vi "testCreateQueues.vi"(8 "error in (no error)":errorcluster) -> (0 "error out":errorcluster)   [LabVIEW 2018]
doc: "Test the createQueues.vi."
uses:
  src/TcpServerBase/TcpServerBase.lvclass
  src/TcpServerBase/TcpServerBase.lvclass/TcpServerBase.ctl
  <vilib>/addons/_JKI Toolkits/Caraya/classes/Assert/Assert Equal Type_Variant.vi
  <vilib>/addons/_JKI Toolkits/Caraya/classes/Test/Test.lvclass
  <vilib>/addons/_JKI Toolkits/Caraya/classes/Assert/Assert.lvclass
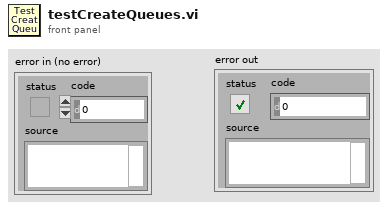
[diagram p1: front panel]
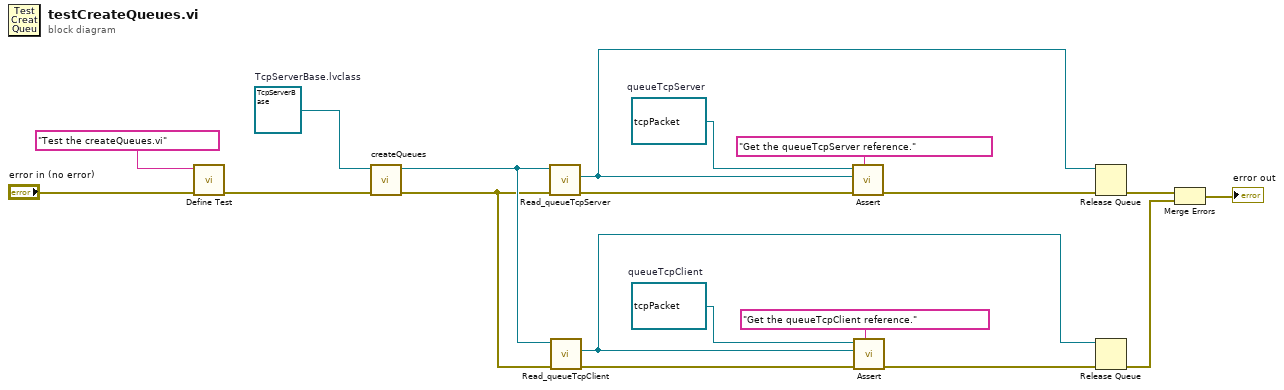
[diagram p0: block diagram]
diagram:
  w1 = refnum<queue> refnum  # queueTcpClient
  w2 = refnum<queue> refnum  # queueTcpServer
  w12 = refnum<class "TcpServerBase.lvclass"> refnum  # TcpServerBase.lvclass
  n1 = call <vilib>:"Define Test.vi"("error in (no error)"="error in (no error)", "Label (VI Title)"="Test the createQueues.vi") -> ("error out"=w11:errorcluster)  [unwired: 9 in]
  n2 = call "createQueues.vi"("error in (no error)"=w11, "tcpServerBase in"=w12) -> ("error out"=w9:errorcluster, "tcpServerBase out"=w10:refnum<class "TcpServerBase.lvclass">)  [unwired: 8 in]
  n3 = call "Read_queueTcpServer.vi"("error in (no error)"=w9, "TcpServerBase in"=w10) -> ("error out"=w8:errorcluster, "queueTcpServer"=w4:refnum<queue>)  [unwired: 7 in, 1 out]
  n4 = call "Read_queueTcpClient.vi"("error in (no error)"=w9, "TcpServerBase in"=w10) -> ("error out"=w7:errorcluster, "queueTcpClient"=w3:refnum<queue>)  [unwired: 7 in, 1 out]
  n5 = call-poly <vilib>:"Assert.vi"("Label"="Get the queueTcpServer reference.", "error in (no error)"=w8, "Y"=w4, "X"=w2) -> ("error out"=w16:errorcluster)  [unwired: 7 in]
  n6 = call-poly <vilib>:"Assert.vi"("Label"="Get the queueTcpClient reference.", "error in (no error)"=w7, "Y"=w3, "X"=w1) -> ("error out"=w15:errorcluster)  [unwired: 7 in]
  n7 = Release Queue(queue=w4, error in (no error)=w16) -> (error out=w6:errorcluster)  [unwired: 1 in, 2 out]
  n8 = Release Queue(queue=w3, error in (no error)=w15) -> (error out=w5:errorcluster)  [unwired: 1 in, 2 out]
  n9 = Merge Errors(w6, w5) -> (→"error out":errorcluster)
